vi "update_map.vi"(10 "New Values":map{string, string}(c390), 11 "Source":map{string, string}(c390)) -> (3 "Updated":map{string, string}(c390))   [LabVIEW 2019, in "Conditional Disable Build Actions.lvlib"]
uses:
  Conditional Disable Build Actions.lvlib
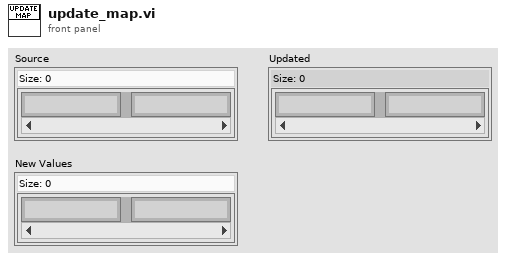
[diagram p1: front panel]
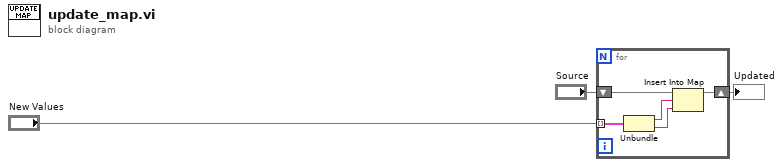
[diagram p0: block diagram]
diagram:
  n1 = for {
    shift-right: [w4] -> w1
    shift-left: "Source" -> [w8]
    tunnel: "New Values" -> [w7] mode=indexing
    n2 = Unbundle(w7) -> ("key"=w6:string, "value"=w5:string)
    n3 = Insert Into Map(map in=w8, key=w6, value=w5) -> (map out=w4:map{string, string})  [unwired: 2 out]
  }
  "Updated" <- w1
